vi "Live window-Set tick boxes.vi"   [LabVIEW 2020]
uses:
  Global Variables/General Globals.vi
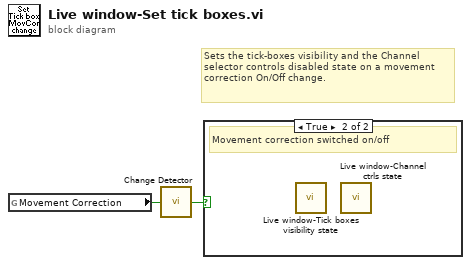
[diagram p0: block diagram]
diagram:
  # "Sets the tick-boxes visibility and the Channel selector controls disabled state on a movement correction On/Off change."
  n1 = global read "General Globals.vi" "Movement Correction"() -> (w1:bool)
  n2 = call <userlib>:"Change Detector.vi"("Value"=w1) -> ("Changed?"=w2:bool)
  n3 = case shown="True" w2 {
    frame False {
      # "Idle"
    }
    frame True {
      # "Movement correction switched on/off"
      n4 = call "Live window-Tick boxes visibility state.vi"() -> ()  [unwired: 11 in, 1 out]
      n5 = call "Live window-Channel ctrls state.vi"() -> ()  [unwired: 12 in]
    }
  }
